vi "dataProcess_power.vi"(0 "reference":refnum<class "OSA.lvclass">, 2 "spectrum x unit (wavenr/cm)":T1, 3 "spectrum y unit (mW pwr absolute)":T2=enum."mW pwr absolute", 4 "yData":sgl[](array[numeric]) format="%.2f", 5 "error in (no error)":errorcluster, 6 "xMin":sgl format="%.2f", 7 "yData length":u32, 8 "xMax":sgl format="%.2f", 9 "xMin power":sgl format="%.2f", 11 "xMax power":sgl format="%.2f") -> (14 "duplicate reference":refnum<class "OSA.lvclass">, 19 "error out":errorcluster)   [LabVIEW 2010, in "OSA.lvclass"]
doc: "This calculates the total optical power in the given spectrum between the points xMin power and xMax power. The X data is format is x min and max, (parameter xMin and xMax). \n\nParameters\n\nxMin, xMax, yData length, spectrum x unit: defines spectrum X-array.\n\nyData, spectrum y unit: defines spectrum Y-array.\n\nxMin power, xMax power: power integration range."
uses:
  OSA.lvclass
  typeDef/spectrum_y_unit.ctl
  typeDef/spectrum_x_unit.ctl
  FTSLib.dll
panel:
  in  "dummy":dbl
  out "result":dbl format="%.2f"
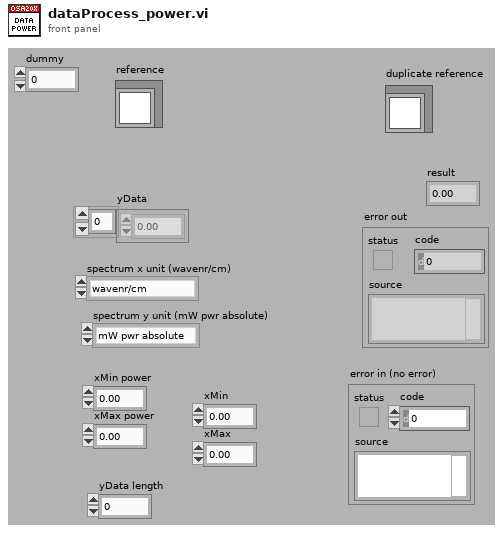
[diagram p1: front panel]
types:
  T1 = typedef "OSA.lvclass/spectrum_x_unit.ctl" = enum16{"wavenr/cm", "THz", "eV", "nm_air", "nm_vac"}
  T2 = typedef "OSA.lvclass/spectrum_y_unit.ctl" = enum16{"dBm pwr absolute", "dBm pwr density", "mW pwr absolute", "mW pwr density"}
  T3 = typedef "OSA.lvclass/ObjectAttributes.ctl" = cluster{"Stop":bool, "dataType":T4, "spectrometerIdx":u16, "buffer size interferogram":i32, "interferogram":cluster{"new":bool, "plot_x_ min":sgl, "plot_x_max":sgl, "plot_y_min":sgl, "plot_y_max":sgl, "Graph Intrfrgrm":T5, "timeStamp":u32, "signal (%)":dbl, "traces":cluster{"idx":u32, "broadBand":bool, "monoChromatic":bool, "peakToPeakSignal":dbl, "peakToPeakPos":dbl}[], "traces idx last":i32}, "spectrum":cluster{"new":bool, "plot_x_min":sgl, "plot_x_max":sgl, "plot_unit_x":T1, "plot_unit_y":T6, "plot_y_min":sgl, "plot_y_max":sgl, "Graph Spectrum":T5, "timeStamp":u32, "X_VAL_OPTIONS":enum16{"MIN_MAX", "ARRAY"}, "traces":cluster{"idx":u32}[], "traces idx last":i32}, "Thorlabs_OSA_64.lvclass:queue_action.ctlqueue ref":refnum<queue>, "action":T7, "plot zoom step":dbl, "buffer semaphore":T8, "acq stopped":bool, "dataType active":T4, "temperature (degr C)":sgl, "pressure (hPa)":sgl, "rel humidity (%)":sgl, "settings":cluster{"resolution":T9, "sensitivity":T10, "Average":bool, "average nr":u32, "apodisation":T11, "acq delay (ms)":u32, "airMesure":T12, "wmtr on":bool, "intfgrm_smooth_width":u16, "intfgrm_smooth_nrOfPasses":u16, "intfgrm_smooth":T13, "phaseCorrection":T14, "zeroFill":u8, "spectr_smooth":T13, "spectr_smooth_width":u16, "spectr_smooth_nrOfPasses":u16, "resolution (/cm)":sgl, "REF wavelength, (nm)":dbl, "gain_idx":u16, "gainAuto":bool, "gain_relative":dbl, "PD sensitivity mode":T15, "PD senseMode implemented":bool, "SensorTemperature implemented":bool, "SensorPressure implemented":bool, "SensorHumidity implemented":bool}, "peaks position":sgl[], "peaks width":sgl[], "peaks height":sgl[], "peaks max nr":u32, "peaks latest nr":i32, "peaks new":bool, "power":dbl, "power new":bool, "path":string, "wavelength (WNr)":dbl, "wavelength new":bool, "buffer size spectrum":i32, "status":string, "VI reference":refnum<vi>, "funcPointer":u64, "libraryPointer":u64, "singleAcquisition":bool, "coherenceLength (cm)":dbl, "coherenceLength new":bool, "spectrometer model":string, "spectrometer serial nr":string, "peaks thld left":sgl[], "peaks thld right":sgl[], "coherenceLength error (cm)":dbl, "ADC bits":u16, "peaks position centroid":sgl[], "peaks height centroid":sgl[], "OSA series":T16, "channel index":u16, "channel index stiched":u16, "spectrum channel type":T17}
  T4 = typedef "OSA.lvclass/acq_dataType.ctl" = enum16{"none", "interferogram", "spectrum"}
  T5 = typedef "OSA.lvclass/graph_intensity.ctl" = refnum<vi>
  T6 = typedef "OSA.lvclass/y_unit.ctl" = enum16{"ADC counts", "dBm pwr absolute", "dBm pwr density", "mW pwr absolute", "mW pwr density"}
  T7 = typedef "OSA.lvclass/queue_action.ctl" = enum16{"none", "stop", "GUI_plotInterferogram", "GUI_plotSpectrum", "GUI_plotInterferogramRescale", "GUI_plotSpectrumRescale", "GUI_plotInterferogramReset", "GUI_plotSpectrumReset", "GUI_plotInterferogramAutoScaleY", "GUI_plotSpectrumAutoScaleY", "GUI_plotInterferogramZoomOut", "GUI_plotSpectrumZoomOut", "GUI_plotInterferogramPane", "GUI_plotSpectrumPane", "GUI_plotInterferogramZoomMouse", "GUI_plotSpectrumZoomMouse", "ENVIRONMENT temperature", "ENVIRONMENT pressure", "MODE_resolution set", "MODE_resolution get", "MODE_sensitivity set", "MODE_sensitivity get", "MODE_PDTemperature set", "MODE_PDTemperature get", "REBOOT/RESET firmware", "ACQASYNC_acquireSingleSpectrum", "ACQASYNC_continuous start", "ACQASYNC_continuous stop\n", "ACQASYNC_get last interferogram", "ACQASYNC_get last spectrum", "ACQASYNC_get last waveNr", "ACQOPT_interferogram smoothing set", "ACQOPT_interferogram smoothing get", "ACQOPT_spectrum smoothing set", "ACQOPT_spectrum smoothing get", "ACQOPT_apodisation type set", "ACQOPT_apodisation type get", "ACQOPT_phase correction type set", "ACQOPT_phase correction type get", "ACQOPT_acqIntervall_set", "ACQOPT_acqIntervall_get", "ACQOPT_average spectrum set", "ACQOPT_average spectrum get", "ACQOPT_rolling average set", "ACQOPT_rolling average get", "ACQOPT_zero fill factor set", "ACQOPT_zero fill factor get", "ACQOPT_cycle counting set", "ACQOPT_cycle counting get", "ACQOPT_air measure option set", "ACQOPT_air measure option get", "ACQOPT_gainLevel auto get", "ACQOPT_gainLevel auto set", "ACQOPT_gainLevel get", "ACQOPT_gainLevel set", "ACQOPT_getAll", "INSTRUMENT_PROPERTY_range_WaveNr_min", "INSTRUMENT_PROPERTY_range_WaveNr_max", "INSTRUMENT_PROPERTY_reference_wavelength_cm^-1", "INSTRUMENT_PROPERTY_samplesPerRefPeriod", "INSTRUMENT_PROPERTY_resolution_waveNrPercm", "INSTRUMENT_PROPERTY_availableGainLevels", "INSTRUMENT_PROPERTY_status", "CONVERT", "ANALYSE_POWER", "ANALYSE_PEAKS", "ANALYSE_WAVELENGTH", "ANALYSE_SPECTRUM", "ANALYSE_INTERFEROGRAM", "ANALYSE_COHERENCE_LENGTH", "MATH", "MATH_power", "MATH_peaks", "FILE", "miscellaneous"}
  T8 = typedef "Semaphore RefNum" = refnum<k1>
  T9 = typedef "OSA.lvclass/resolution.ctl" = enum16{"low", "high"}
  T10 = typedef "OSA.lvclass/sensitivityMode.ctl" = enum16{"low", "low medium", "high medium", "high"}
  T11 = typedef "OSA.lvclass/apodisation.ctl" = enum16{"NONE", "NORTON_BEER_WEAK", "NORTON_BEER_MEDIUM", "NORTON_BEER_STRONG", "TRIANGULAR", "COSINE", "HANN", "HAMMING", "BLACKMANHARRIS3", "BLACKMANHARRIS4", "GAUSSIAN"}
  T12 = typedef "OSA.lvclass/airMeasure.ctl" = enum16{"TEMPERATURE", "PRESSURE"}
  T13 = typedef "OSA.lvclass/smoothing.ctl" = enum16{"NONE", "BINOMIAL", "SAVITSKY_GOLAY", "FOURIER", "MOVING_AVERAGE", "GAUSSIAN"}
  T14 = typedef "OSA.lvclass/phaseCorrection.ctl" = enum16{"NONE", "MERTZ", "FORMAN", "MERTZ_FILE", "FORMAN_FILE", "FUTURE COMP."}
  T15 = typedef "OSA.lvclass/PDTemperatureMode.ctl" = enum16{"cool: better sensitivity/noise floor", "warm: extended wl range"}
  T16 = typedef "OSA.lvclass/OSA_series.ctl" = enum16{"OSA200", "OSA300", "UNKNOWN"}
  T17 = typedef "OSA.lvclass/channelType_spectrum.ctl" = enum16{"SINGLE CHANNEL", "STICHED"}
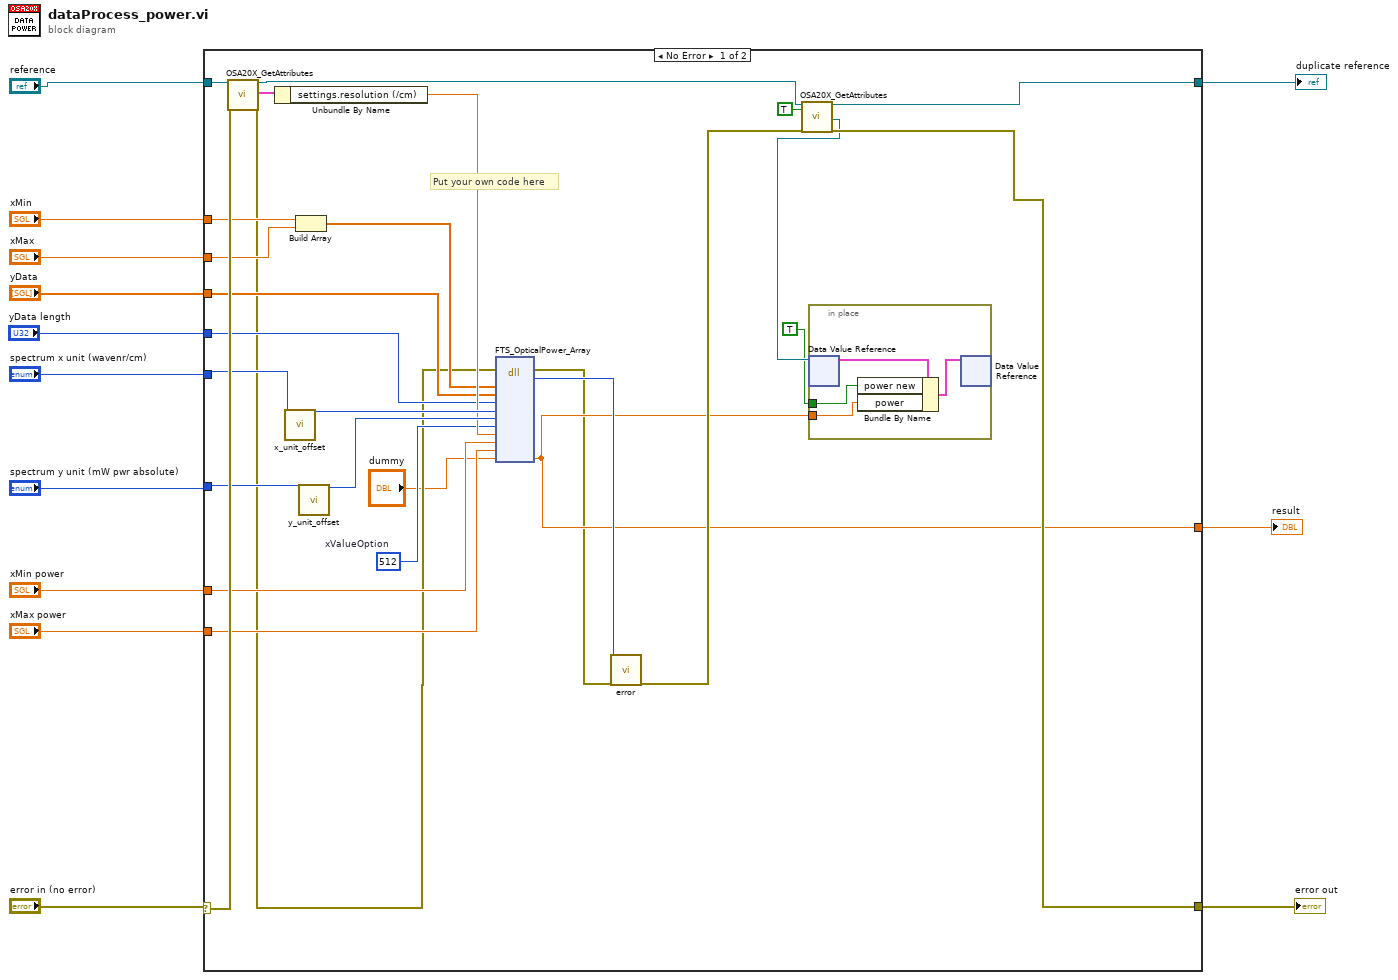
[diagram p0: block diagram]
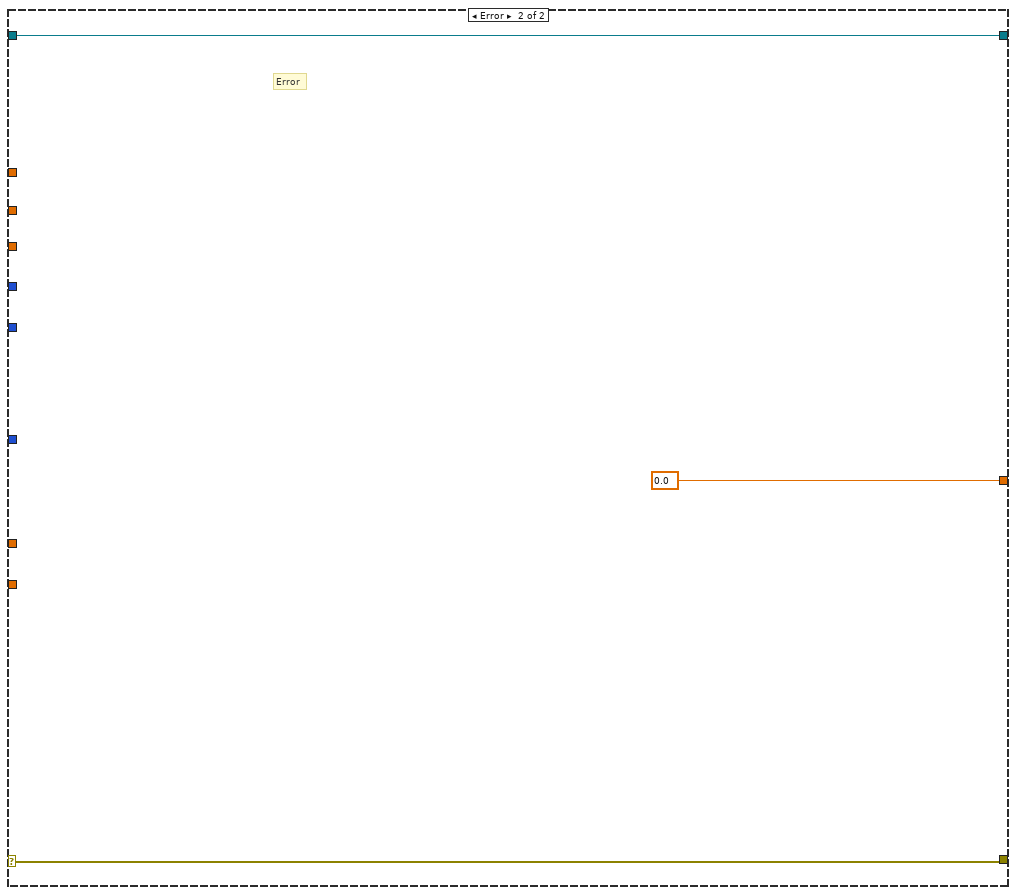
[diagram p2: hidden frame]
diagram:
  n1 = case shown="No Error" "error in (no error)" {
    selector: "error in (no error)" -> [w40 w47]
    tunnel: [w27 w47] -> w13
    tunnel: "reference" -> [w41 w48]
    tunnel: [w29 w48] -> w10
    tunnel: "spectrum y unit (mW pwr absolute)" -> [w38 _]
    tunnel: "yData" -> [w23 _]
    tunnel: "spectrum x unit (wavenr/cm)" -> [w35 _]
    tunnel: "xMin power" -> [w34 _]
    tunnel: "xMax power" -> [w33 _]
    tunnel: [w17 0.0 ("result")] -> w4
    tunnel: "xMin" -> [w26 _]
    tunnel: "xMax" -> [w25 _]
    tunnel: "yData length" -> [w22 _]
    frame No Error {
      w31 = u32 512  # xValueOption
      # "Put your own code here"
      n2 = call "OSA20X_GetAttributes.vi"("reference in"=w41, "error in (no error)"=w40) -> ("reference out"=w30:refnum<class "OSA.lvclass">, "Data"=w20:T3, "error out"=w16:errorcluster)  [unwired: 14 in, 1 out]
      n3 = Unbundle By Name(w20) -> ("settings.resolution (/cm)"=w32:sgl)
      n4 = call "x_unit_offset.vi"("spectrum x unit (wavenr/cm)"=w35) -> ("xUnit val"=w36:i32)  [unwired: 18 in]
      n5 = Build Array(w26, w25) -> (w24:sgl[])
      n6 = call "y_unit_offset.vi"("spectrum y unit (mW pwr absolute)"=w38) -> ("yUnit val"=w37:i32)  [unwired: 18 in]
      n7 = dll-call lib="FTSLib.dll" fn="FTS_OpticalPower_Array"(error in=w16, "xData"=w24, "yData"=w23, "length"=w22, "xAxisUnit"=w36, "yAxisUnit"=w37, "xValueOption"=w31, "resolution_wnr"=w32, "xMin"=w34, "xMax"=w33, "result"="dummy") -> (error out=w15:errorcluster, "return type"=w39:i32, "result"=w17:dbl)  [unwired: 11 in, 1 out]
      n8 = call "error.vi"("result code"=w39, "error in (no error)"=w15) -> ("error out"=w28:errorcluster)  [unwired: 15 in, 2 out]
      n9 = call "OSA20X_GetAttributes.vi"("reference in"=w30, "OnlyGetDvrReference(False)"=TRUE, "error in (no error)"=w28) -> ("reference out"=w29:refnum<class "OSA.lvclass">, "DataRef"=w19:refnum<data-value>, "error out"=w27:errorcluster)  [unwired: 13 in, 1 out]
      n10 = in-place {
        in-place-border: TRUE ("peaks new") -> [w44]
        in-place-border: w17 -> [w43]
        n11 = in-place-dvr #1(w19) -> (w45:T3)  [unwired: 1 out]
        n12 = Bundle By Name(cluster=w45, "power new"=w44, "power"=w43) -> (w42:T3)
        n13 = in-place-dvr #1(w42) -> ()  [unwired: 2 out]
      }
    }
    frame Error {
      # "Error"
    }
  }
  "error out" <- w13
  "duplicate reference" <- w10
  "result" <- w4
